vi "Saturate Phi.vi"(7 "HS?":bool, 11 "Phi In":dbl) -> (3 "Phi Out":dbl)   [LabVIEW 2018]
panel:
  out "Phi":cluster{"Phi In":dbl, "Phi In":dbl}(graph)
  out "Diff Phi":dbl(graph)
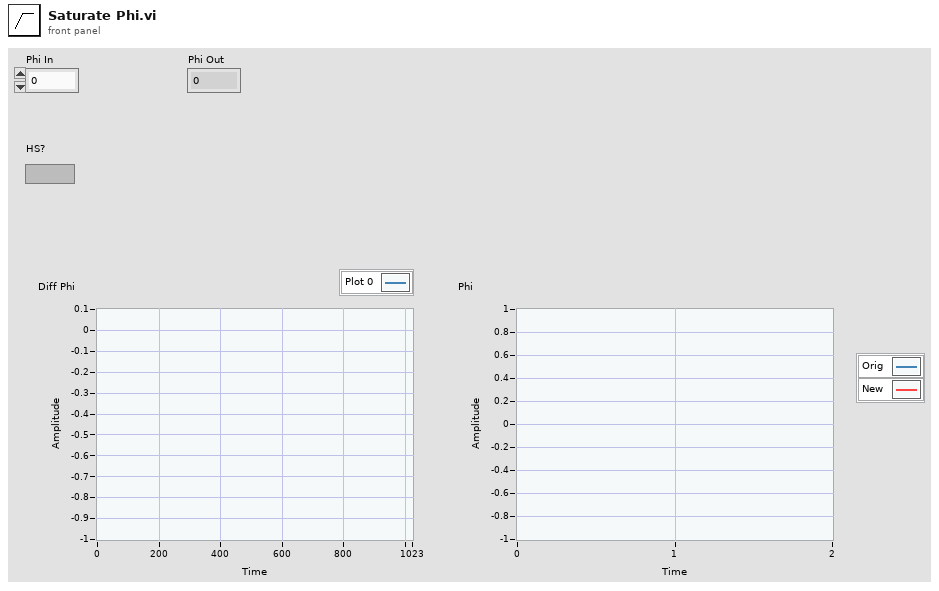
[diagram p1: front panel]
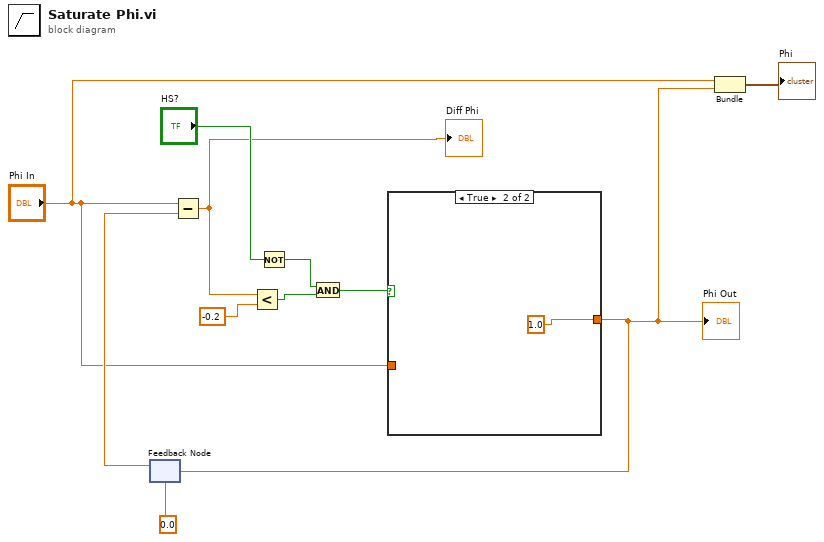
[diagram p0: block diagram]
diagram:
  n1 = feedback #1(0.0 ("initial condition")) -> (w4:dbl)
  n2 = Subtract(x="Phi In", y=w4) -> (x-y=w5:dbl)
  "Diff Phi" <- w5
  n3 = Less?(x=w5, y=-0.2) -> (x < y?=w9:bool)
  n4 = Not(x="HS?") -> (.not. x?=w7:bool)
  n5 = And(x=w7, y=w9) -> (x .and. y?=w8:bool)
  n6 = case shown="True" w8 {
    tunnel: [w12 1.0] -> w2
    tunnel: "Phi In" -> [w12 _]
    frame False {
    }
    frame True {
    }
  }
  "Phi Out" <- w2
  n7 = feedback-in #1(w2) -> ()
  n8 = Bundle("Phi In"="Phi In", "Phi In"=w2) -> (→"Phi":cluster{"Phi In":dbl, "Phi In":dbl})  [unwired: 1 in]
